vi "InsertDevicePanel.vi"(0 "Communication in":refnum<class "Microscope.lvclass">, 5 "Panel":string, 9 "VI Refnum":refnum<vi>, 11 "error in (no error)":errorcluster) -> (4 "Communication out":refnum<class "Microscope.lvclass">, 15 "error out":errorcluster)   [LabVIEW 2020, in "Microscope.lvlib" / "Microscope.lvclass"]
uses:
  Microscope.lvclass
  ViewController/Microscope Controller Messages/InsertPanelToMainframe Msg/InsertPanelToMainframe Msg.lvclass/InsertPanelToMainframe Msg.ctl
  <vilib>/ActorFramework/Message Enqueuer/Message Enqueuer.lvclass/Message Enqueuer.ctl
  <vilib>/ActorFramework/Message Enqueuer/Enqueue.vi
  ViewController/Microscope Controller Messages/InsertPanelToMainframe Msg/InsertPanelToMainframe Msg.lvclass
  C:/Program Files/National Instruments/LabVIEW 2020/vi.lib/ActorFramework/Message/Message.lvclass
  <vilib>/ActorFramework/Message Priority Queue/Priority Enqueue.vi
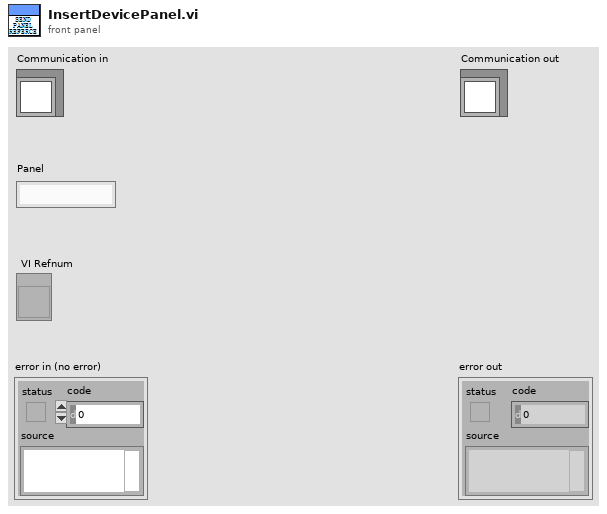
[diagram p1: front panel]
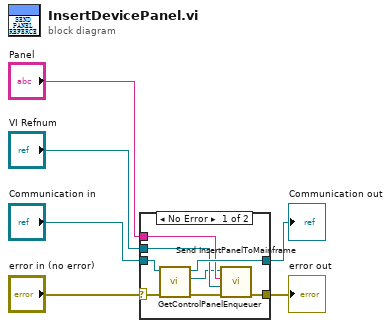
[diagram p0: block diagram]
diagram:
  n1 = case shown="No Error" "error in (no error)" {
    selector: "error in (no error)" -> [w12 w16]
    tunnel: [w9 w16] -> w5
    tunnel: [w13 w15] -> w3
    tunnel: "Communication in" -> [w14 w15]
    tunnel: "VI Refnum" -> [w10 _]
    tunnel: "Panel" -> [w11 _]
    frame No Error {
      n2 = call-dynamic "GetControlPanelEnqueuer.vi"("error in (no error)"=w12, "GRMActor in"=w14) -> ("error out"=w8:errorcluster, "ControlViewEnqueuer"=w7:refnum<class "Message Enqueuer.lvclass">, "GRMActor out"=w13:refnum<class "Microscope.lvclass">)  [unwired: 7 in]
      n3 = call "Send InsertPanelToMainframe.vi"("error in (no error)"=w8, "VI Refnum"=w10, "Sub Panel"=w11, "Message Enqueuer"=w7) -> ("error out"=w9:errorcluster)  [unwired: 6 in, 1 out]
    }
    frame Error {
    }
  }
  "error out" <- w5
  "Communication out" <- w3
